vi "timer11.vi"() -> ()   [LabVIEW 2019]
uses:
  Program Files (x86)/National Instruments/LabVIEW 2019/project/EN1Course-master (12)/EN1Course-master/_Subs/SystemLink/SL_Subs/SL_XControl.xctl
  <vilib>/httpClient/POSTBuffer.vi
  Program Files (x86)/National Instruments/LabVIEW 2019/project/EN1Course-master (12)/EN1Course-master/_Subs/SystemLink/SL_Subs/SystemLink_Write_Number.vi
  <vilib>/httpClient/LabVIEWHTTPClient.lvlib
panel:
  in  "timer sec":T1(xcontrol)={"Tag"="Timer", "Type"="U_INT64", "Data"="11"}
  in  "timer minutes":T1(xcontrol)={"Tag"="Timer1", "Type"="U_INT64", "Data"="0"}
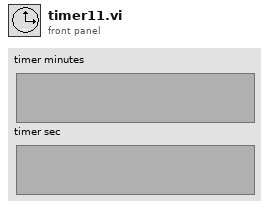
[diagram p1: front panel]
types:
  T1 = cluster{"Tag":string, "Type":string, "Data":string}
  T2 = enum16{"Button", "Clear", "Timer", "Circuit", "Stop"}
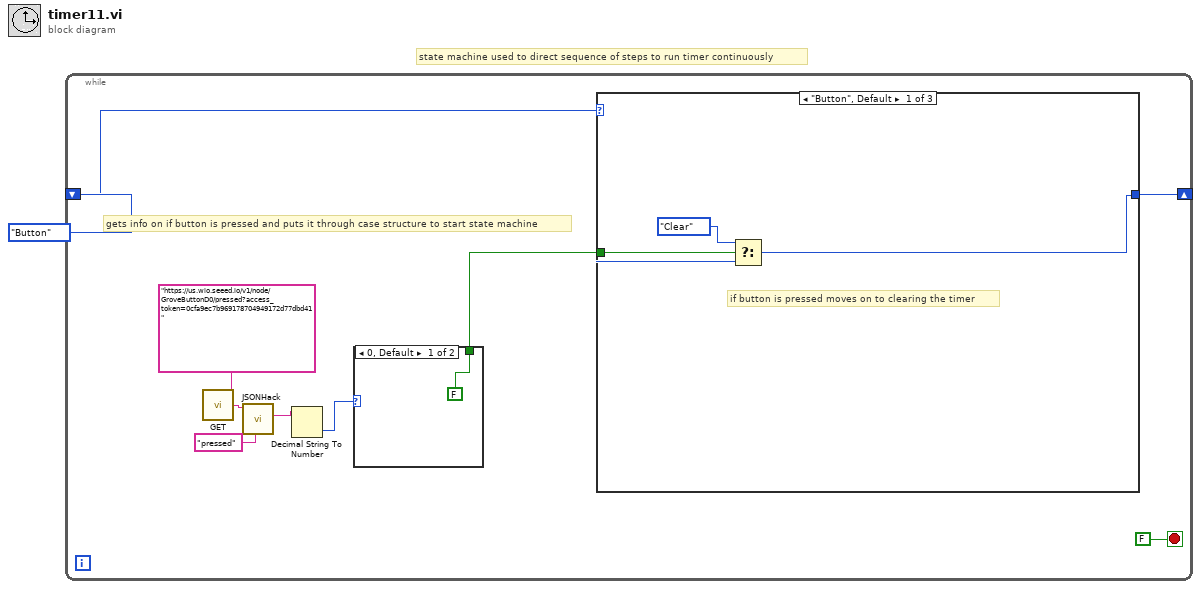
[diagram p0: block diagram]
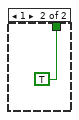
[diagram p2: hidden frame]
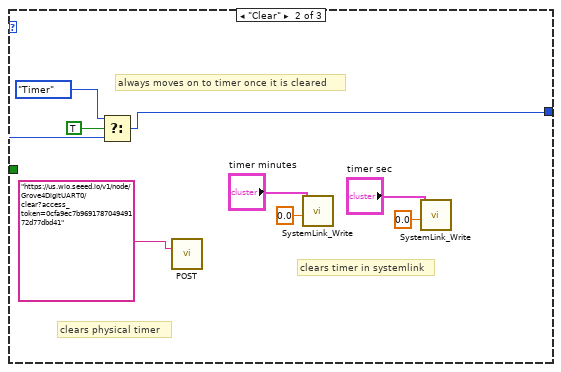
[diagram p3: hidden frame]
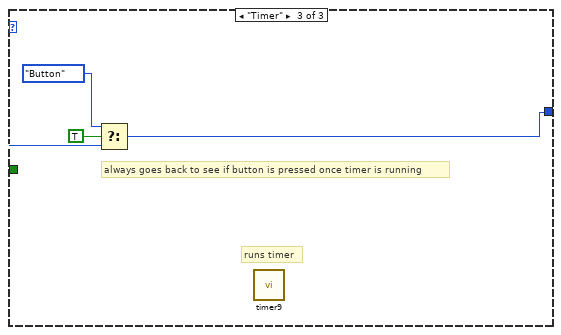
[diagram p4: hidden frame]
diagram:
  # "state machine used to direct sequence of steps to run timer continuously"
  n1 = while {
    shift-right: [w3] -> _
    shift-left: enum16{"Button", "Clear", "Timer"}."Button" -> [w10]
    stop <- FALSE stop-if-true
    # "gets info on if button is pressed and puts it through case structure to start state machine"
    n2 = call <vilib>:"GET.vi"("url"="https://us.wio.seeed.io/v1/node/GroveButtonD0/pressed?access_token=0cfa9ec7b969178704949172d77dbd41") -> ("body"=w8:string)  [unwired: 11 in, 3 out]
    n3 = call "JSONHack.vi"("search name"="pressed", "JSON in"=w8) -> ("Property (str)"=w9:string)  [unwired: 6 in, 3 out]
    n4 = Decimal String To Number(string=w9) -> (number=w5:i32)  [unwired: 2 in, 1 out]
    n5 = case shown="0, Default" w5 {
      tunnel: [FALSE ("s") TRUE ("s")] -> w4
      frame 0, Default {
      }
      frame 1 {
      }
    }
    n6 = case shown="\"Button\", Default" w10 {
      selector: w10 -> [w16 w25 w29]
      tunnel: w4 -> [w14 _ _]
      tunnel: [w13 w21 w26] -> w3
      frame "Button", Default {
        # "if button is pressed moves on to clearing the timer"
        n7 = Select(t=T2."Clear", s=w14, f=w16) -> (s? t:f=w13:T2)
      }
      frame "Clear" {
        # "always moves on to timer once it is cleared"
        # "clears timer in systemlink"
        # "clears physical timer"
        n8 = Select(t=T2."Timer", s=TRUE, f=w25) -> (s? t:f=w21:T2)
        n9 = call-poly <vilib>:"POST.vi"("url"="https://us.wio.seeed.io/v1/node/Grove4DigitUART0/clear?access_token=0cfa9ec7b969178704949172d77dbd41") -> ()  [unwired: 11 in, 4 out]
        n10 = call-poly "SystemLink_Write.vi"("Numeric"=0.0, "SL_XControl"="timer minutes") -> ()  [unwired: 10 in]
        n11 = call-poly "SystemLink_Write.vi"("Numeric"=0.0, "SL_XControl"="timer sec") -> ()  [unwired: 10 in]
      }
      frame "Timer" {
        # "always goes back to see if button is pressed once timer is running"
        # "runs timer"
        n12 = Select(t=T2."Button", s=TRUE, f=w29) -> (s? t:f=w26:T2)
        n13 = call "timer9.vi"() -> ()  [unwired: 11 in, 1 out]
      }
    }
  }
